vi "hardwareRunExample.vi"() -> ()   [LabVIEW 2026]
uses:
  <vilib>/DAQmx/write.llb/DAQmx Write (Digital 1D Bool 1Chan 1Samp).vi
  <vilib>/DAQmx/read.llb/DAQmx Read (Analog 2D DBL NChan NSamp).vi
  <vilib>/DAQmx/read.llb/DAQmx Read (Digital 1D Bool 1Chan 1Samp).vi
  <vilib>/DAQmx/create/channels.llb/DAQmx Create Channel (AI-Voltage-Basic).vi
  <vilib>/DAQmx/configure/timing.llb/DAQmx Timing (Sample Clock).vi
  <vilib>/DAQmx/create/channels.llb/DAQmx Create Channel (DI-Digital Input).vi
  <vilib>/DAQmx/create/channels.llb/DAQmx Create Channel (DO-Digital Output).vi
  <vilib>/DAQmx/miscellaneous.llb/DAQmx Fill In Error Info.vi
panel:
  in  "data 3":bool[](array[boolean])
  out "data 2":bool[](array[boolean])
  out "1/x":dbl
  out "data":dbl[][](array[numeric]) format="%0.2f"
  in  "Boolean":bool
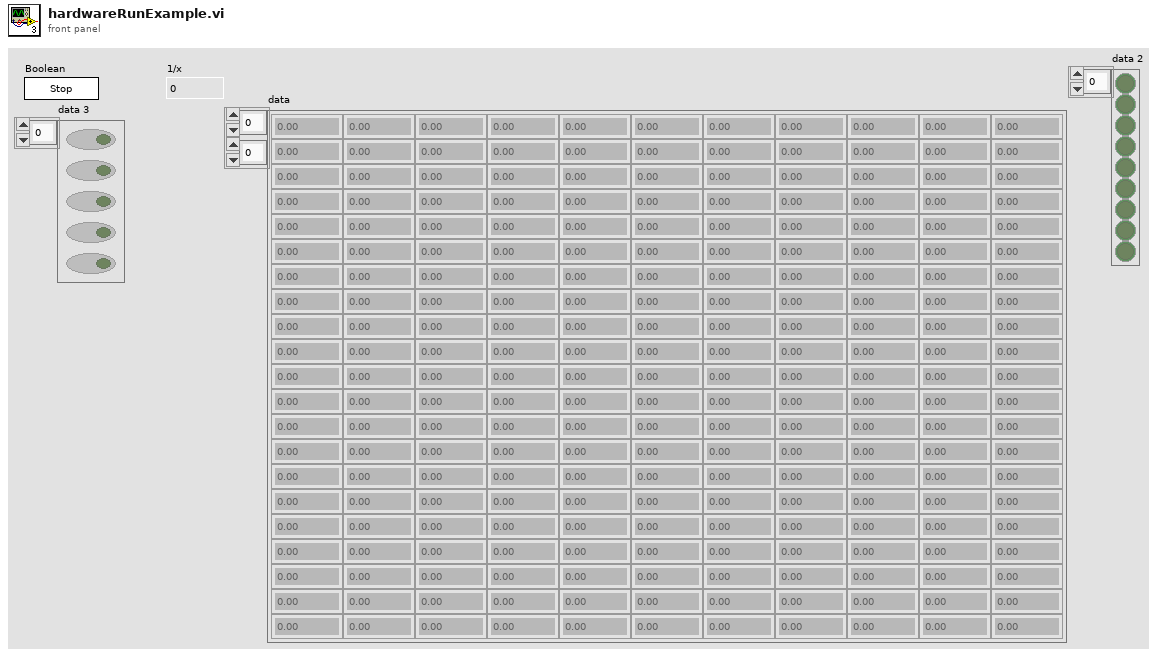
[diagram p1: front panel]
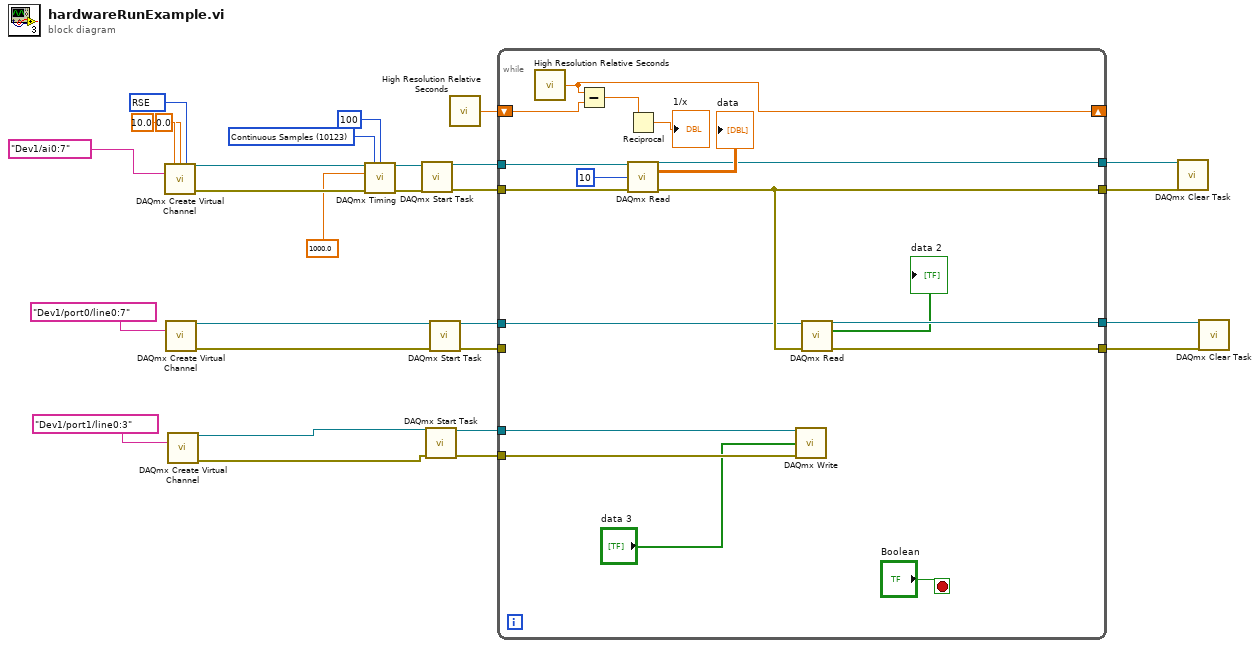
[diagram p0: block diagram]
diagram:
  w22 = 10123 items=["Finite Samples"=10178, "Continuous Samples"=10123, "Hardware Timed Single Point"=12522] ("sample mode")
  w26 = 10083 items=["Default"=-1, "RSE"=10083, "NRSE"=10078, "Differential"=10106, "Pseudodifferential"=12529] ("input terminal configuration")
  n1 = call-poly <vilib>:"DAQmx Create Virtual Channel.vi"("maximum value"=10.0, "minimum value"=0.0, "input terminal configuration"=w26, "physical channels"=tag "Dev1/ai0:7") -> ("task out"=w23:refnum<k21>, "error out"=w24:errorcluster)  [unwired: 10 in]
  n2 = call-poly <vilib>:"DAQmx Create Virtual Channel.vi"("lines"=tag "Dev1/port0/line0:7") -> ("task out"=w11:refnum<k21>, "error out"=w10:errorcluster)  [unwired: 13 in]
  n3 = call-poly <vilib>:"DAQmx Create Virtual Channel.vi"("lines"=tag "Dev1/port1/line0:3") -> ("task out"=w4:refnum<k21>, "error out"=w3:errorcluster)  [unwired: 13 in]
  n4 = call-poly <vilib>:"DAQmx Timing.vi"("task/channels in"=w23, "sample mode"=w22, "samples per channel"=100, "rate"=1000.0, "error in"=w24) -> ("task out"=w19:refnum<k21>, "error out"=w18:errorcluster)  [unwired: 9 in]
  n5 = call <vilib>:"DAQmx Start Task.vi"("task/channels in"=w19, "error in"=w18) -> ("task out"=w17:refnum<k21>, "error out"=w16:errorcluster)  [unwired: 12 in]
  n6 = call <vilib>:"DAQmx Start Task.vi"("task/channels in"=w4, "error in"=w3) -> ("task out"=w2:refnum<k21>, "error out"=w1:errorcluster)  [unwired: 12 in]
  n7 = call <vilib>:"DAQmx Start Task.vi"("task/channels in"=w11, "error in"=w10) -> ("task out"=w8:refnum<k21>, "error out"=w9:errorcluster)  [unwired: 12 in]
  n8 = call <vilib>:"High Resolution Relative Seconds.vi"() -> ("relative seconds"=w13:dbl)
  n9 = while {
    tunnel: w17 -> [w46]
    tunnel: w16 -> [w45]
    tunnel: [w42] -> w15
    tunnel: [w36] -> w14
    shift-right: [w38] -> _
    shift-left: w13 -> [w40]
    tunnel: w9 -> [_]
    tunnel: w8 -> [w35]
    tunnel: [w34] -> w7
    tunnel: [w33] -> w6
    tunnel: w2 -> [w31]
    tunnel: w1 -> [w30]
    stop <- "Boolean" stop-if-true
    n10 = call <vilib>:"High Resolution Relative Seconds.vi"() -> ("relative seconds"=w38:dbl)
    n11 = Subtract(x=w38, y=w40) -> (x-y=w39:dbl)
    n12 = Reciprocal(x=w39) -> (1/x=→"1/x":dbl)
    n13 = call-poly <vilib>:"DAQmx Read.vi"("task/channels in"=w46, "number of samples per channel"=10, "error in"=w45) -> ("task out"=w42:refnum<k21>, "data"=→"data":dbl[][], "error out"=w36:errorcluster)  [unwired: 10 in]
    n14 = call-poly <vilib>:"DAQmx Write.vi"("task/channels in"=w31, "data"="data 3", "error in"=w30) -> ()  [unwired: 10 in, 3 out]
    n15 = call-poly <vilib>:"DAQmx Read.vi"("task/channels in"=w35, "error in"=w36) -> ("task out"=w33:refnum<k21>, "data"=→"data 2":bool[], "error out"=w34:errorcluster)  [unwired: 11 in]
  }
  n16 = call <vilib>:"DAQmx Clear Task.vi"("task in"=w15, "error in"=w14) -> ()  [unwired: 13 in, 1 out]
  n17 = call <vilib>:"DAQmx Clear Task.vi"("task in"=w6, "error in"=w7) -> ()  [unwired: 13 in, 1 out]
